vi "Write to BC.vi"(8 "error in (no error)":errorcluster, 9 "data words":u16[](array[numeric]), 10 "number of words":u16, 11 "rt transfer handle":u64) -> (0 "error out":errorcluster)   [LabVIEW 2023, in "Ballard MIL-STD-1553 Engine Support.lvlib" / "Implementation.lvlib" / "Tx Execution Unit.lvclass"]
uses:
  Tx Execution Unit.lvclass
  <instrlib>/BTI1553Lib/BTI1553LV.lvlib
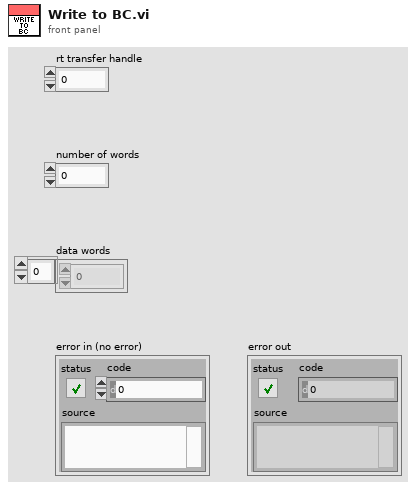
[diagram p1: front panel]
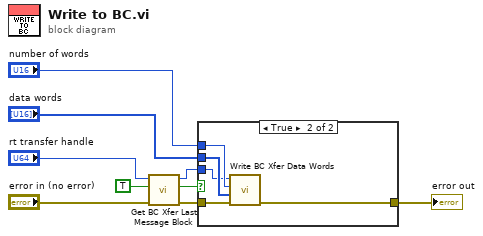
[diagram p0: block diagram]
diagram:
  n1 = call <instrlib>:"Get BC Xfer Last Message Block.vi"("error in (no error)"="error in (no error)", "clear hit?"=TRUE, "bc transfer handle in"="rt transfer handle") -> ("error out"=w3:errorcluster, "was hit?"=w2:bool, "bc transfer handle out"=w5:u64)  [unwired: 5 in, 1 out]
  n2 = case shown="True" w2 {
    tunnel: [w10 w15] -> w9
    tunnel: "number of words" -> [_ w14]
    tunnel: "data words" -> [_ w13]
    tunnel: w5 -> [_ w12]
    tunnel: w3 -> [w10 w11]
    frame False {
    }
    frame True {
      n3 = call <instrlib>:"Write BC Xfer Data Words.vi"("error in (no error)"=w11, "data words"=w13, "data word count in"=w14, "bc transfer handle in"=w12) -> ("error out"=w15:errorcluster)  [unwired: 5 in, 2 out]
    }
  }
  "error out" <- w9
